vi "Get Audio File Info (Core).vi"(8 "error in (no error)":errorcluster, 11 "Path In":string) -> (0 "error out":errorcluster, 1 "Audio File Info":T2, 2 "PCM Frame Length":u64, 3 "Path Out":string, 4 "Codec":T1)   [LabVIEW 2020, in "G-Audio.lvlib"]
doc: "Retrieve audio file information. Some codecs (mp3) require the entire file be parsed to accurately determine the length, which can take time for very large files.\n\nSupported codecs: flac, mp3, ogg (vorbis), and wav."
uses:
  G-Audio.lvlib
  Controls/Audio File Info.ctl
  Controls/Audio File Codec.ctl
  <vilib>/Utility/error.llb/Error Cluster From Error Code.vi
  lib/g_audio_32.dll
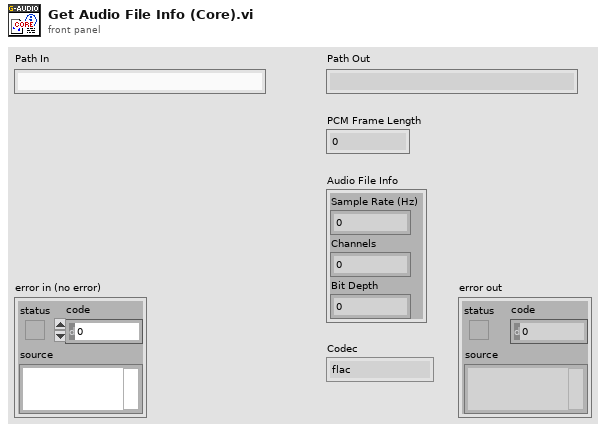
[diagram p1: front panel]
types:
  T1 = typedef "G-Audio.lvlib/Audio File Codec.ctl" = enum16{"flac", "mp3", "vorbis", "wav", "unsupported"}
  T2 = typedef "G-Audio.lvlib/Audio File Info.ctl" = cluster{"Sample Rate (Hz)":u32, "Channels":u32, "Bit Depth":u32}
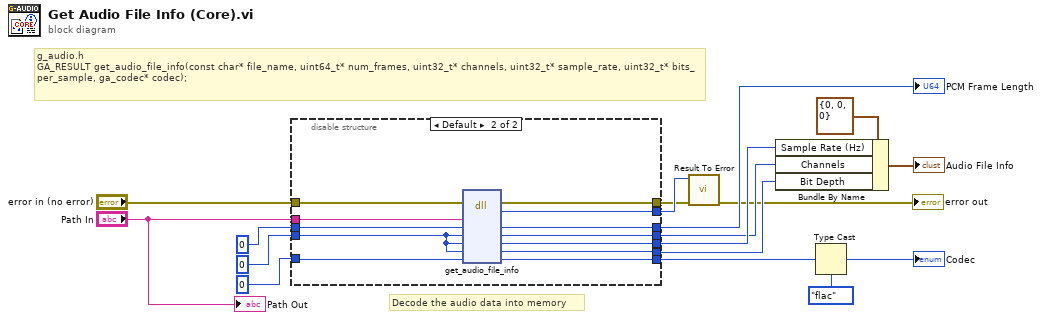
[diagram p0: block diagram]
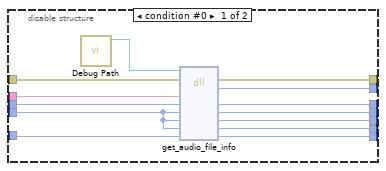
[diagram p2: hidden frame]
diagram:
  # "g_audio.h\nGA_RESULT get_audio_file_info(const char* file_name, uint64_t* num_frames, uint32_t* channels, uint32_t* sample_rate, uint32_t* bits_per_sample, ga_codec* codec);"
  # "Decode the audio data into memory"
  n1 = disable-structure shown="Default" {
    disable-tunnel: "error in (no error)" -> [w30 w42]
    disable-tunnel: [w28 w40] -> w15
    disable-tunnel: [w27 w39] -> w11
    disable-tunnel: [w26 w38] -> w12
    disable-tunnel: "Path In" -> [w25 w37]
    disable-tunnel: [w29 w41] -> w8
    disable-tunnel: u32 0 ("num_samples") -> [w23 w35]
    disable-tunnel: u64 0 ("num_samples") -> [w24 w36]
    disable-tunnel: [w22 w34] -> w13
    disable-tunnel: [w21 w33] -> w9
    disable-tunnel: [w19 w31] -> w6
    disable-tunnel: u16 0 ("num_samples") -> [w18 w32]
    frame condition #0 {
      n2 = call "Debug Path.vi"() -> ("Debug Path"=w20:path)  [unwired: 11 in]
      n3 = dll-call lib="?" fn="get_audio_file_info"(path in=w20, error in=w30, "file_name"=w25, "num_frames"=w24, "channels"=w23, "sample_rate"=w23, "bits_per_sample"=w23, "codec"=w18) -> (error out=w29:errorcluster, "result"=w21:i32, "num_frames"=w28:u64, "channels"=w27:u32, "sample_rate"=w26:u32, "bits_per_sample"=w22:u32, "codec"=w19:u16)  [unwired: 2 in, 1 out]
    }
    frame condition #1 (active) {
      n4 = dll-call lib="C:/github/dataflowg/g-audio/src/LabVIEW/G-Audio/lib/g_audio_*.*" fn="get_audio_file_info"(error in=w42, "file_name"=w37, "num_frames"=w36, "channels"=w35, "sample_rate"=w35, "bits_per_sample"=w35, "codec"=w32) -> (error out=w41:errorcluster, "result"=w33:i32, "num_frames"=w40:u64, "channels"=w39:u32, "sample_rate"=w38:u32, "bits_per_sample"=w34:u32, "codec"=w31:u16)  [unwired: 3 in, 1 out]
    }
  }
  "PCM Frame Length" <- w15
  n5 = call "Result To Error.vi"("error in (no error)"=w8, "Result Code"=w9) -> ("error out"=→"error out":errorcluster)  [unwired: 9 in]
  n6 = Bundle By Name(cluster=T2 {"Sample Rate (Hz)"=0, "Channels"=0, "Bit Depth"=0} ("Audio File Info"), "Sample Rate (Hz)"=w12, "Channels"=w11, "Bit Depth"=w13) -> (→"Audio File Info":T2)
  n7 = Type Cast(type=Audio_File_Codec."flac" ("Codec"), x=w6) -> (*(type *) &x=→"Codec":T1)
  "Path Out" <- "Path In"
